vi "Trigger.vi"(8 "Error In":errorcluster, 11 "reference in":refnum<class "Clippy.lvclass">) -> (0 "Error Out":errorcluster, 3 "reference out":refnum<class "Clippy.lvclass">)   [LabVIEW 2020, in "Clippy.lvclass"]
doc: "This method gets called every time the trigger elaps"
uses:
  Clippy.lvclass
  AnimationTypes.ctl
  <vilib>/numeric/Random Number (Range) U64.vi
  <vilib>/numeric/sub_Random U32.vi
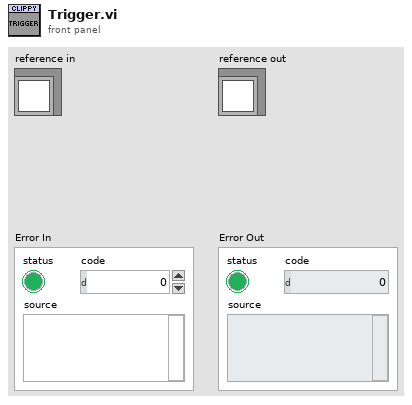
[diagram p1: front panel]
types:
  T1 = typedef "Clippy.lvclass/AnimationTypes.ctl" = enum16{"Congratulate", "LookRight", "SendMail", "Thinking", "Explain", "IdleRopePile", "IdleAtom", "Print", "Hide", "GetAttention", "Save", "GetTechy", "GestureUp", "Idle1_1", "Processing", "Alert", "LookUpRight", "IdleSideToSide", "GoodBye", "LookLeft", "IdleHeadScratch", "LookUpLeft", "CheckingSomething", "Hearing_1", "GetWizardy", "IdleFingerTap", "GestureLeft", "Wave", "GestureRight", "Writing", "IdleSnooze", "LookDownRight", "GetArtsy", "Show", "LookDown", "Searching", "EmptyTrash", "Greeting", "LookUp", "GestureDown", "RestPose", "IdleEyeBrowRaise", "LookDownLeft"}
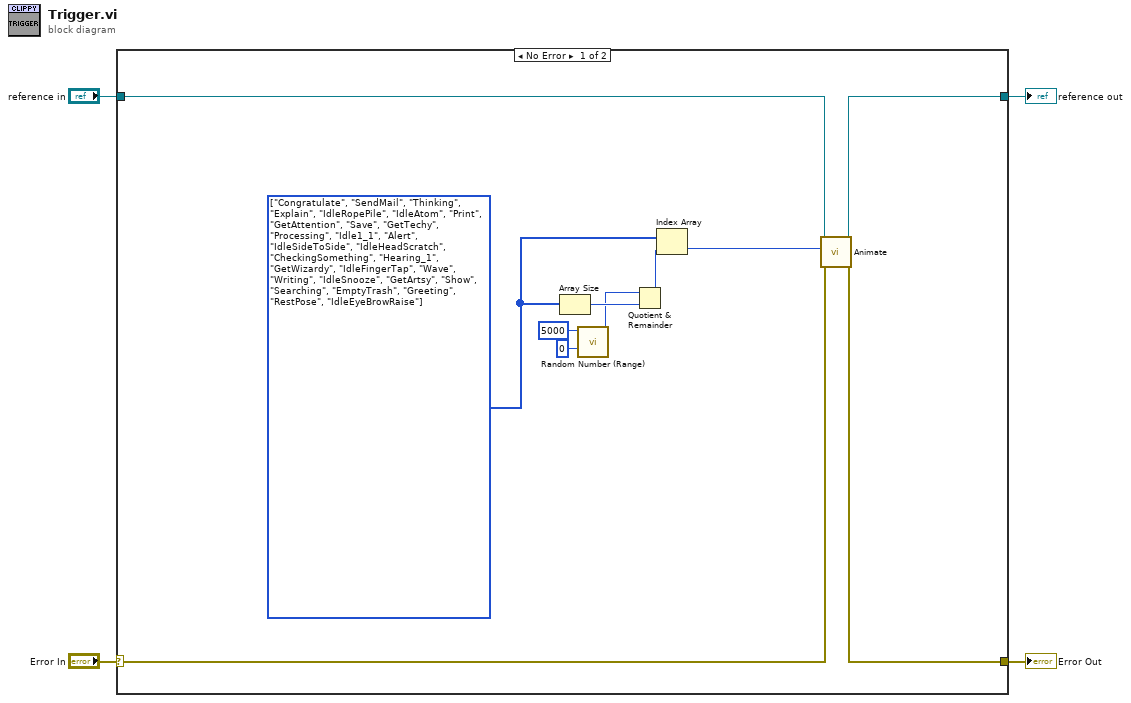
[diagram p0: block diagram]
diagram:
  n1 = case shown="No Error" "Error In" {
    selector: "Error In" -> [w6 w17]
    tunnel: [w5 w17] -> w3
    tunnel: [w7 w16] -> w1
    tunnel: "reference in" -> [w8 w16]
    frame No Error {
      w12 = T1[] [enum."Congratulate", enum."SendMail", enum."Thinking", enum."Explain", enum."IdleRopePile", enum."IdleAtom", enum."Print", enum."GetAttention", enum."Save", enum."GetTechy", enum."Processing", enum."Idle1_1", enum."Alert", enum."IdleSideToSide", enum."IdleHeadScratch", enum."CheckingSomething", enum."Hearing_1", enum."GetWizardy", enum."IdleFingerTap", enum."Wave", enum."Writing", enum."IdleSnooze", enum."GetArtsy", enum."Show", enum."Searching", enum."EmptyTrash", enum."Greeting", enum."RestPose", enum."IdleEyeBrowRaise"] items=["Congratulate", "LookRight", "SendMail", "Thinking", "Explain", "IdleRopePile", "IdleAtom", "Print", "Hide", "GetAttention", "Save", "GetTechy", "GestureUp", "Idle1_1", "Processing", "Alert", "LookUpRight", "IdleSideToSide", "GoodBye", "LookLeft", "IdleHeadScratch", "LookUpLeft", "CheckingSomething", "Hearing_1", "GetWizardy", "IdleFingerTap", "GestureLeft", "Wave", "GestureRight", "Writing", "IdleSnooze", "LookDownRight", "GetArtsy", "Show", "LookDown", "Searching", "EmptyTrash", "Greeting", "LookUp", "GestureDown", "RestPose", "IdleEyeBrowRaise", "LookDownLeft"] ("Array")
      n2 = Array Size(array=w12) -> (size(s)=w13:i32)
      n3 = call-poly <vilib>:"Random Number (Range).vi"("lower bound (0)"=u64 0, "upper bound (100)"=u64 5000) -> ("number"=w9:u64)  [unwired: 9 in]
      n4 = Quotient & Remainder(x=w9, y=w13) -> (x-y*floor(x/y)=w11:u64)  [unwired: 1 out]
      n5 = Index Array(array=w12, index=w11) -> (element=w10:T1)
      n6 = call-dynamic "Animate.vi"("Error In"=w6, "Animation"=w10, "reference in"=w8) -> ("Error Out"=w5:errorcluster, "reference out"=w7:refnum<class "Clippy.lvclass">)  [unwired: 7 in]
    }
    frame Error {
    }
  }
  "Error Out" <- w3
  "reference out" <- w1
